vi "5_5.vi"() -> ()   [LabVIEW 2018]
uses:
  <vilib>/gmath/NI_Gmath.lvlib
panel:
  out "观测次数m":i32
  out "理论最佳误码率":dbl
  in  "观测时刻（0-1）":dbl[](array[numeric])=[0.0, 0.0909090909, 0.1818181818, 0.27272727272, 0.36363636363, 0.454545454545, 0.545454545454, 0.6363636363636, 0.72727272727, 0.81818181818, 0.909090909, 1.0]
  out "噪声标准差":dbl
  out "设计误码率":ext
  out "理论最优门限":dbl
  out "先验概率P(H1)":dbl
  in  "先验概率P(H0)":dbl=0.5
  in  "噪声方差":dbl=0.5
  in  "样本数":u64=1000000
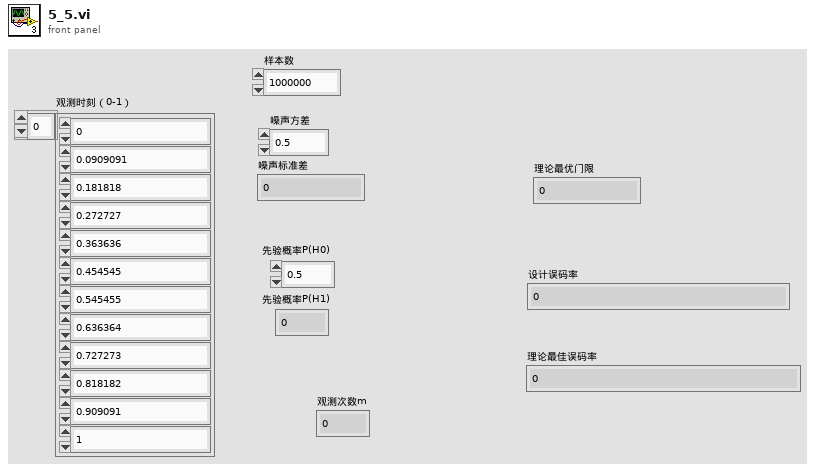
[diagram p1: front panel]
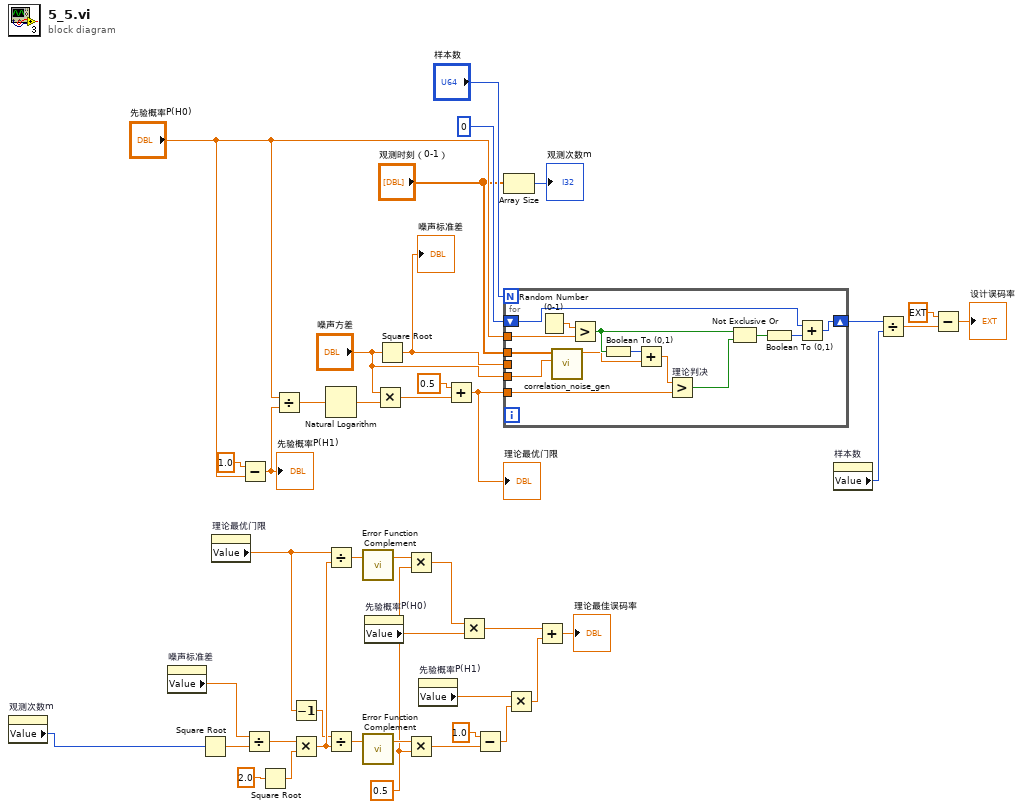
[diagram p0: block diagram]
diagram:
  w17 = 0.5 ("y")
  n1 = property on="观测次数m" class="DigNum (严格)"() -> ("Value"=w1:i32)  [unwired: 2 in, 2 out]
  n2 = property on="噪声标准差" class="DigNum (严格)"() -> ("Value"=w6:dbl)  [unwired: 2 in, 2 out]
  n3 = Square Root(x=w1) -> (sqrt(x)=w9:dbl)
  n4 = property on="理论最优门限" class="DigNum (严格)"() -> ("Value"=w7:dbl)  [unwired: 2 in, 2 out]
  n5 = Subtract(x=1.0, y="先验概率P(H0)") -> (x-y=w35:dbl)
  "先验概率P(H1)" <- w35
  n6 = Divide(x=w6, y=w9) -> (x/y=w8:dbl)
  n7 = Square Root(x=2.0) -> (sqrt(x)=w24:dbl)
  n8 = Divide(x="先验概率P(H0)", y=w35) -> (x/y=w40:dbl)
  n9 = Decrement(x=w7) -> (x-1=w22:dbl)
  n10 = Multiply(x=w8, y=w24) -> (x*y=w23:dbl)
  n11 = Natural Logarithm(1:w40) -> (0:w39:dbl)
  n12 = Divide(x=w7, y=w23) -> (x/y=w21:dbl)
  n13 = Divide(x=w22, y=w23) -> (x/y=w20:dbl)
  n14 = call <vilib>:"Error Function Complement.vi"("x"=w21) -> ("1 - erf(x)"=w18:dbl)  [unwired: 2 in]
  n15 = call <vilib>:"Error Function Complement.vi"("x"=w20) -> ("1 - erf(x)"=w19:dbl)  [unwired: 2 in]
  n16 = property on="先验概率P(H0)" class="DigNum (严格)"() -> ("Value"=w3:dbl)  [unwired: 2 in, 2 out]
  n17 = Multiply(x="噪声方差", y=w39) -> (x*y=w38:dbl)
  n18 = Square Root(x="噪声方差") -> (sqrt(x)=w29:dbl)
  "噪声标准差" <- w29
  n19 = Multiply(x=w18, y=w17) -> (x*y=w13:dbl)
  n20 = Multiply(x=w19, y=w17) -> (x*y=w16:dbl)
  n21 = property on="先验概率P(H1)" class="DigNum (严格)"() -> ("Value"=w2:dbl)  [unwired: 2 in, 2 out]
  n22 = Add(x=0.5, y=w38) -> (x+y=w33:dbl)
  "理论最优门限" <- w33
  n23 = Multiply(x=w13, y=w3) -> (x*y=w10:dbl)
  n24 = Subtract(x=1.0, y=w16) -> (x-y=w12:dbl)
  n25 = Array Size(array="观测时刻（0-1）") -> (size(s)=→"观测次数m":i32)
  n26 = for {
    N: "样本数" -> [_]
    tunnel: "先验概率P(H0)" -> [w55]
    tunnel: w33 -> [w54]
    shift-right: [w52] -> w28
    shift-left: u64 0 ("元素") -> [w50]
    tunnel: w29 -> [_]
    tunnel: "噪声方差" -> [w46]
    tunnel: "观测时刻（0-1）" -> [w45]
    n27 = Random Number (0-1)() -> (number: 0 to 1=w56:dbl)
    n28 = call "correlation_noise_gen.vi"("噪声方差"=w46, "观测时刻（0-1）"=w45) -> ("平均观测噪声"=w44:dbl)  [unwired: 9 in]
    n29 = Greater?(x=w56, y=w55) -> (0:w47:bool)
    n30 = Boolean To (0,1)(Boolean=w47) -> (0, 1=w49:i16)
    n31 = Add(x=w49, y=w44) -> (x+y=w43:dbl)
    n32 = Greater? "理论判决"(x=w43, y=w54) -> (0:w53:bool)
    n33 = Not Exclusive Or(1:w53, 2:w47) -> (0:w48:bool)
    n34 = Boolean To (0,1)(Boolean=w48) -> (0, 1=w51:i16)
    n35 = Add(x=w50, y=w51) -> (x+y=w52:u64)
  }
  n36 = Multiply(x=w2, y=w12) -> (x*y=w11:dbl)
  n37 = Add(x=w10, y=w11) -> (x+y=→"理论最佳误码率":dbl)
  n38 = property on="样本数" class="DigNum (严格)"() -> ("Value"=w27:u64)  [unwired: 2 in, 2 out]
  n39 = Divide(x=w28, y=w27) -> (x/y=w32:dbl)
  n40 = Subtract(x=ext 1.0, y=w32) -> (x-y=→"设计误码率":ext)
